vi "benchmark-memory.vi"() -> ()   [LabVIEW 2020]
uses:
  <vilib>/numeric/Random Number (Range) DBL.vi
panel:
  out "processed":i32
  out "wfmg":dbl[][](graph)
  in  "iterations":i32=1000000
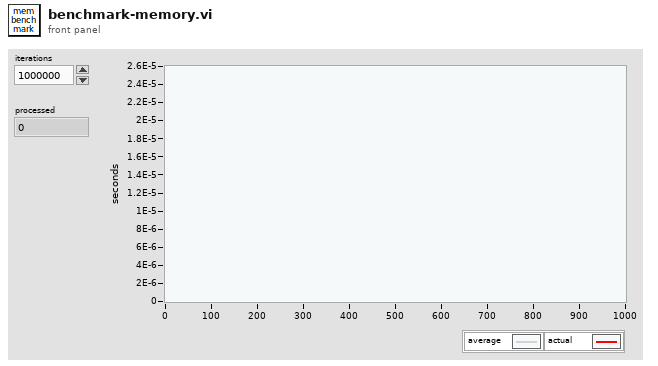
[diagram p1: front panel]
types:
  T1 = typedef "metadata.ctl" = cluster{"worker ID":u32, "min (s)":dbl, "max (s)":dbl, "mean (s)":dbl, "duration (s)":dbl}
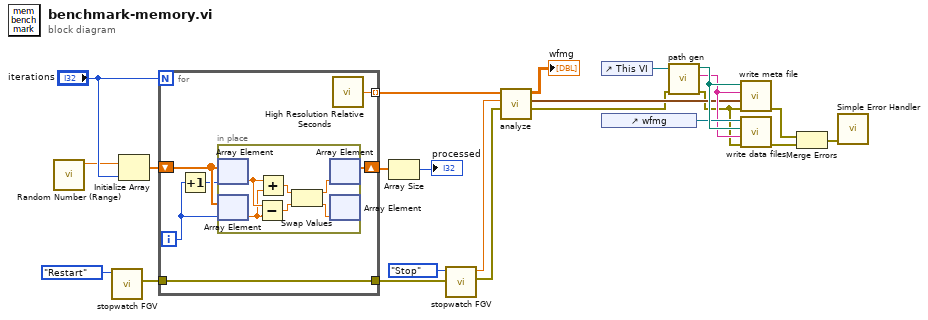
[diagram p0: block diagram]
diagram:
  n1 = call-poly <vilib>:"Random Number (Range).vi"() -> ("number"=w22:dbl)  [unwired: 11 in]
  n2 = call "stopwatch FGV.vi"("state"=enum16{"Restart", "Stop"}."Restart") -> ("error out"=w12:errorcluster)  [unwired: 9 in, 1 out]
  n3 = Initialize Array(w22, "iterations") -> (w21:dbl[])
  n4 = for {
    N: "iterations" -> [_]
    shift-right: [w29] -> w4
    shift-left: w21 -> [w28]
    tunnel: [w25] -> w8 mode=indexing
    tunnel: w12 -> [w24]
    tunnel: [w24] -> w11
    i -> [w26]
    n5 = Increment(x=w26) -> (x+1=w27:i32)
    n6 = in-place {
      n7 = in-place-array #1(w28, w27) -> (w32:dbl)
      n8 = in-place-array #2(w28, w26) -> (w31:dbl)
      n9 = Subtract(x=w32, y=w31) -> (x-y=w33:dbl)
      n10 = Add(x=w32, y=w31) -> (x+y=w30:dbl)
      n11 = Swap Values(12:w30, 14:w33) -> (1:w35:dbl, 3:w34:dbl)  [unwired: 1 in]
      n12 = in-place-array #1(w35) -> (w29:dbl[])  [unwired: 1 out]
      n13 = in-place-array #2(w34) -> ()  [unwired: 2 out]
    }
    n14 = call <vilib>:"High Resolution Relative Seconds.vi"() -> ("relative seconds"=w25:dbl)
  }
  n15 = Array Size(array=w4) -> (size(s)=→"processed":i32)
  n16 = call "stopwatch FGV.vi"("error in"=w11, "state"=enum16{"Restart", "Stop"}."Stop") -> ("error out"=w6:errorcluster, "duration (s)"=w7:dbl)  [unwired: 8 in]
  n17 = call "analyze.vi"("error in"=w6, "duration (s)"=w7, "relative seconds"=w8) -> ("error out"=w2:errorcluster, "metadata"=w5:T1, "data"=→"wfmg":dbl[][])  [unwired: 6 in]
  n18 = control-ref of="This VI"() -> (w13:refnum<vi>)
  n19 = control-ref of="wfmg"() -> (w16:refnum<vi>)
  n20 = call "path gen.vi"("error in"=w2, "Calling VI"=w13) -> ("error out"=w1:errorcluster, "basename"=w15:string, "output folder"=w19:path)  [unwired: 7 in]
  n21 = call "write meta file.vi"("error in"=w1, "metadata"=w5, "file basename"=w15, "output folder"=w19) -> ("error out"=w17:errorcluster)  [unwired: 7 in]
  n22 = call "write data files.vi"("error in"=w1, "file basename"=w15, "output folder"=w19, "WaveformGraph in"=w16) -> ("error out"=w18:errorcluster)  [unwired: 7 in]
  n23 = Merge Errors(w17, w18) -> (w20:errorcluster)
  n24 = call <vilib>:"Simple Error Handler.vi"("error in (no error)"=w20) -> ()  [unwired: 4 in, 5 out]
